vi "CheckMasterConnection.vi"(3 "Master IP":string="Master IP") -> (0 "error out":errorcluster, 1 "Master There?":bool)   [LabVIEW 2012]
doc: "Returns true if it was able to open a connection to the ROS Master"
uses:
  _ROSDefinition.vi
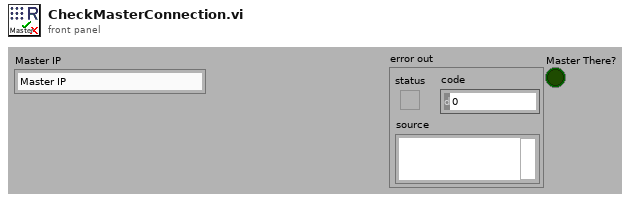
[diagram p1: front panel]
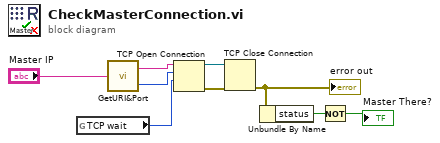
[diagram p0: block diagram]
diagram:
  n1 = global read "_ROSDefinition.vi" "TCP wait"() -> (w1:i32)
  n2 = call "GetURI&Port.vi"("URI in"="Master IP") -> ("Port"=w7:u16, "URI"=w8:string)
  n3 = TCP Open Connection(address=w8, remote port or service name=w7, timeout ms (60000)=w1) -> (connection ID=w5:refnum<k5>, error out=w6:errorcluster)  [unwired: 2 in]
  n4 = TCP Close Connection(connection ID=w5, error in (no error)=w6) -> (error out=w4:errorcluster)  [unwired: 1 in, 1 out]
  "error out" <- w4
  n5 = Unbundle By Name(w4) -> ("status"=w3:bool)
  n6 = Not(x=w3) -> (.not. x?=→"Master There?":bool)
